vi "AddTextLineToListBox.vi"(8 "error in (no error)":errorcluster, 9 "String2":string, 10 "String":string, 11 "ListBox in":refnum<vi>) -> (0 "error out":errorcluster)   [LabVIEW 2023]
doc: "This VI adds a line made out of timestamp+String+String2 (unless they are both empty) into ListBox and clips End of ListBox if bigger than MaxSize (1000)."
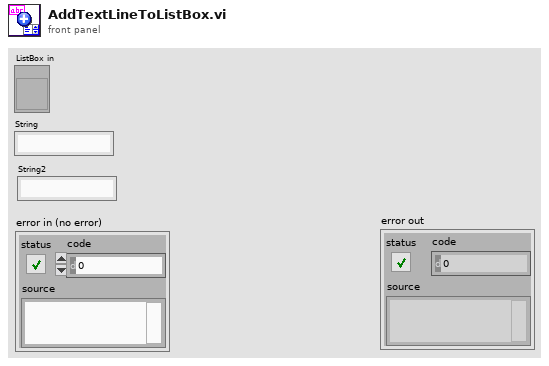
[diagram p1: front panel]
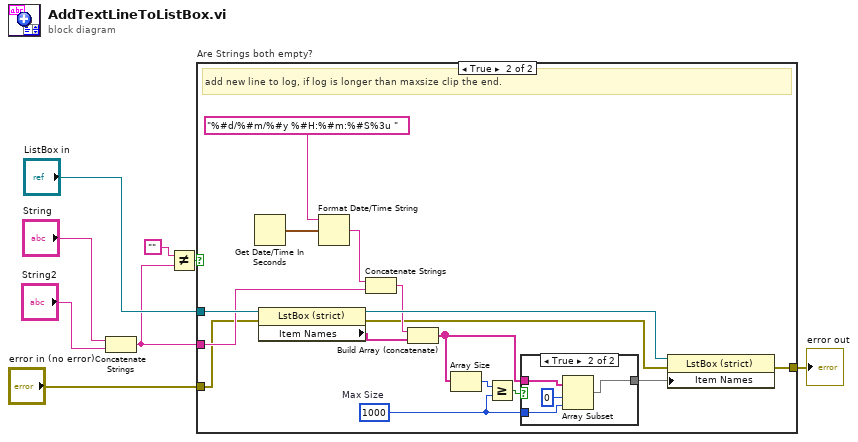
[diagram p0: block diagram]
diagram:
  n1 = Concatenate Strings("String", "String2") -> (w3:string)
  n2 = Not Equal?(x="" ("Empty String Constant"), y=w3) -> (x != y?=w4:bool)
  n3 = case "Are Strings both empty?" shown="True" w4 {
    tunnel: w3 -> [_ w17]
    tunnel: "ListBox in" -> [_ w23]
    tunnel: [w9 w11] -> w2
    tunnel: "error in (no error)" -> [w9 w10]
    frame False {
    }
    frame True {
      w21 = 1000  # Max Size
      # "add new line to log, if log is longer than maxsize clip the end."
      n4 = Get Date/Time In Seconds() -> (seconds since 1Jan1904=w16:timestamp)
      n5 = property on="Property Node" class="LstBox (strict)"(reference=w23, error in=w10) -> (reference out=w24:refnum<vi>, error out=w12:errorcluster, "Item Names"=w25:string[])
      n6 = Format Date/Time String(time format string (%c)="%#d/%#m/%#y %#H:%#m:%#S%3u ", seconds (now)=w16) -> (date/time string=w14:string)  [unwired: 1 in]
      n7 = Concatenate Strings(w14, w17) -> (w13:string)
      n8 = Build Array (concatenate)(w13, w25) -> (w20:string[])
      n9 = Array Size(array=w20) -> (size(s)=w22:i32)
      n10 = Greater Or Equal?(x=w22, y=w21) -> (x >= y?=w18:bool)
      n11 = case shown="True" w18 {
        tunnel: w21 -> [_ w30]
        tunnel: w20 -> [w26 w28]
        tunnel: [w26 w27] -> w19
        frame False {
        }
        frame True {
          n12 = Array Subset(array=w28, index=0, length=w30) -> (w27:string[])
        }
      }
      n13 = property on="Property Node" class="LstBox (strict)"(reference=w24, error in=w12, "Item Names"=w19) -> (error out=w11:errorcluster)  [unwired: 1 out]
    }
  }
  "error out" <- w2
